vi "Check_Speed_And_Incline.vi"(0 "Total Time":dbl, 5 "Display Speed":dbl, 7 "Display Incline":dbl, 9 "Control Speed":dbl, 11 "Control Incline":dbl, 12 "error in (no error)":errorcluster) -> (4 "Speed":dbl, 6 "Incline":dbl, 14 "error out":errorcluster)   [LabVIEW 2026]
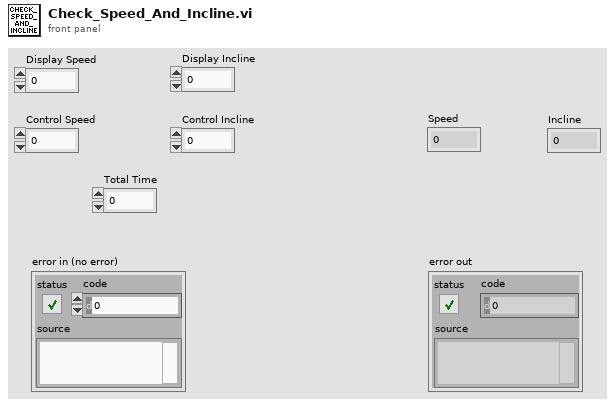
[diagram p1: front panel]
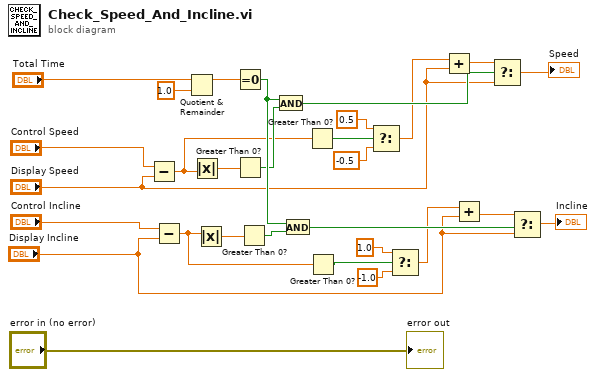
[diagram p0: block diagram]
diagram:
  n1 = Subtract(x="Control Speed", y="Display Speed") -> (x-y=w19:dbl)
  n2 = Subtract(x="Control Incline", y="Display Incline") -> (x-y=w18:dbl)
  n3 = Quotient & Remainder(x="Total Time", y=1.0) -> (x-y*floor(x/y)=w26:dbl)  [unwired: 1 out]
  n4 = Absolute Value(x=w19) -> (abs(x)=w22:dbl)
  n5 = Absolute Value(x=w18) -> (abs(x)=w23:dbl)
  n6 = Equal To 0?(x=w26) -> (x = 0?=w29:bool)
  n7 = Greater Than 0?(x=w22) -> (x > 0?=w27:bool)
  n8 = Greater Than 0?(x=w23) -> (x > 0?=w28:bool)
  n9 = And(x=w29, y=w27) -> (x .and. y?=w8:bool)
  n10 = And(x=w29, y=w28) -> (x .and. y?=w6:bool)
  n11 = Greater Than 0?(x=w19) -> (x > 0?=w16:bool)
  n12 = Greater Than 0?(x=w18) -> (x > 0?=w11:bool)
  n13 = Select(t=0.5, s=w16, f=-0.5 ("t")) -> (s? t:f=w7:dbl)
  n14 = Select(t=1.0, s=w11, f=-1.0 ("t")) -> (s? t:f=w5:dbl)
  n15 = Add(x=w7, y="Display Speed") -> (x+y=w10:dbl)
  n16 = Add(x=w5, y="Display Incline") -> (x+y=w9:dbl)
  n17 = Select(t=w10, s=w8, f="Display Speed") -> (s? t:f=→"Speed":dbl)
  n18 = Select(t=w9, s=w6, f="Display Incline") -> (s? t:f=→"Incline":dbl)
  "error out" <- "error in (no error)"
